vi "ProcessName.vi"() -> (1 "ProcessName":string)   [LabVIEW 2017, in "McsaVirtualChannel.lvlib"]
uses:
  <vilib>/addons/InsightCM/Devices/Shared/Mcsa/McsaVirtualChannel/McsaVirtualChannel.lvlib
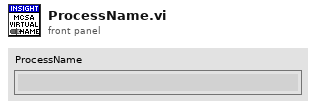
[diagram p1: front panel]
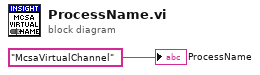
[diagram p0: block diagram]
diagram:
  "ProcessName" <- "McsaVirtualChannel" ("ProcessName")
